vi "DownloadSettings.vi"() -> (1 "Yaxis":dbl[](array[numeric]), 2 "Xaxis":dbl[](array[numeric]), 3 "name":string)   [LabVIEW 2020]
panel:
  in  "Path":path
  in  "Multiplty (Iteration time)":dbl
  in  "OK":bool
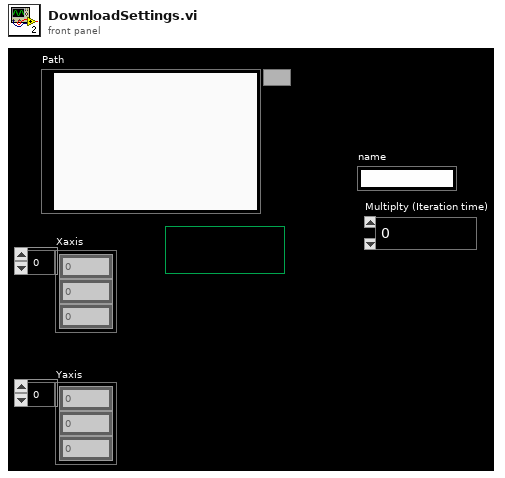
[diagram p1: front panel]
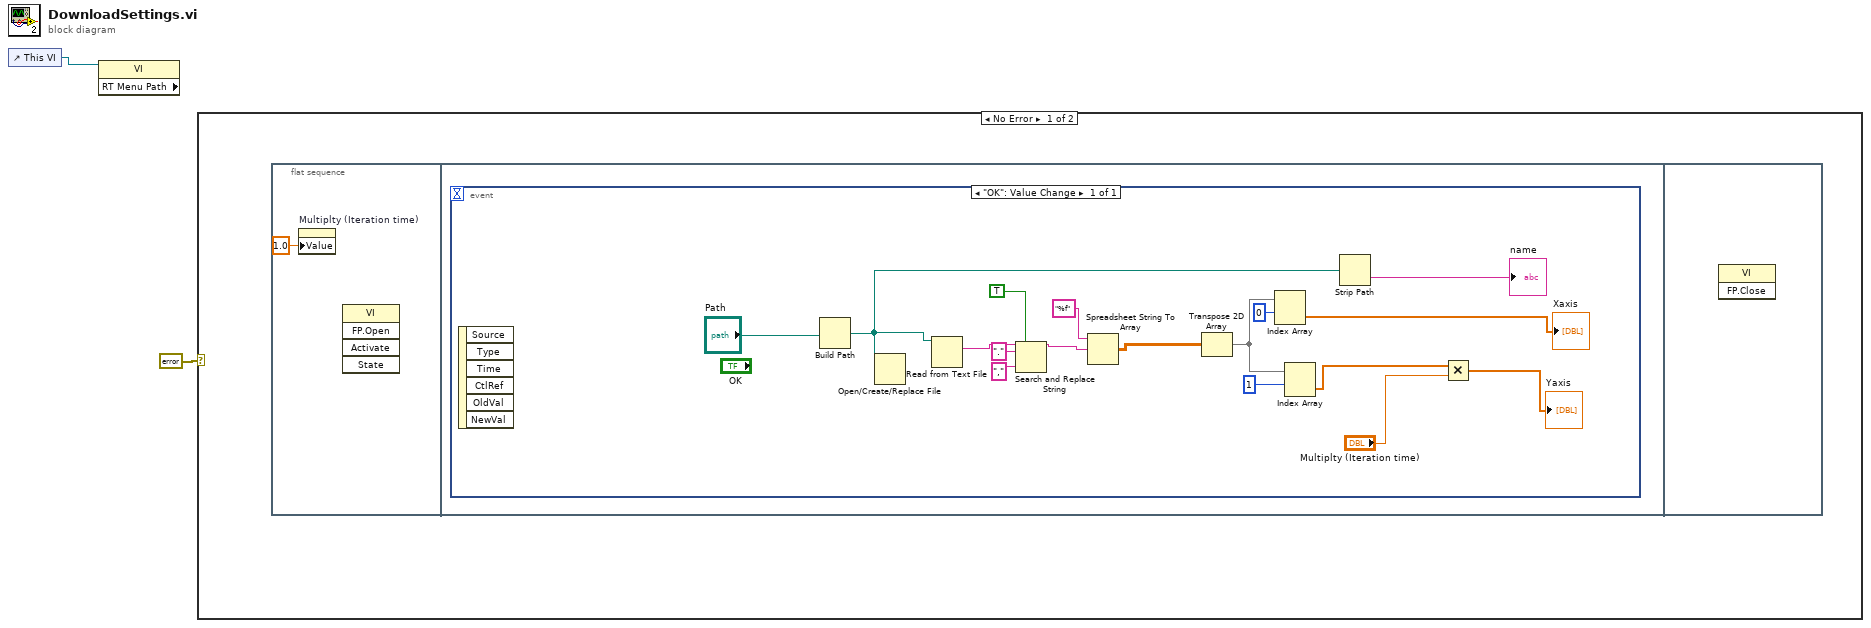
[diagram p0: block diagram]
diagram:
  n1 = control-ref of="This VI"() -> (w1:refnum<vi>)
  n2 = property class="VI" props=["RT Menu Path"](reference=w1) -> ()  [unwired: 1 in, 3 out]
  n3 = case shown="No Error" errorcluster {"status"=FALSE, "code"=0, "source"=""} ("error constant") {
    frame No Error {
      n4 = flat-sequence {
        frame #0 {
          n5 = property on="Multiplty (Iteration time)" class="DigNum (strict)"("Value"=1.0 ("Multiplty (Iteration time)")) -> ()  [unwired: 2 in, 2 out]
          n6 = invoke class="VI" method="FP.Open"() -> ()  [unwired: 5 in, 5 out]
        }
        frame #1 {
          n7 = event shown="[0] \"OK\": Value Change" {
            selector: _ -> [_]
            dyn-events: _ -> [_]
            timeout: _ -> [_]
            event "OK": Value Change {
              n8 = event-data() -> ()  [unwired: 1 in, 6 out]
              n9 = Build Path(name or relative path="Path") -> (appended path=w10:path)  [unwired: 1 in]
              n10 = Open/Create/Replace File(file path (use dialog)=w10) -> ()  [unwired: 5 in, 3 out]
              n11 = Read from Text File(file (use dialog)=w10) -> (text=w16:string)  [unwired: 3 in, 3 out]
              n12 = Search and Replace String(replace all?=TRUE ("replace all? (F)"), input string=w16, search string=".", replace string="," ("replace string (\"\")")) -> (result string=w12:string)  [unwired: 4 in, 3 out]
              n13 = Spreadsheet String To Array(format string="%f", spreadsheet string=w12) -> (array=w11:dbl[][])  [unwired: 2 in]
              n14 = Transpose 2D Array(2D array=w11) -> (transposed array=w18:dbl[][])
              n15 = Index Array(array=w18, index (row)=0) -> (element=→"Xaxis":dbl[])  [unwired: 1 in]
              n16 = Index Array(array=w18, index (row)=1) -> (element=w9:dbl[])  [unwired: 1 in]
              n17 = Strip Path(path=w10) -> (name=→"name":string)  [unwired: 1 out]
              n18 = Multiply(x=w9, y="Multiplty (Iteration time)") -> (x*y=→"Yaxis":dbl[])
            }
          }
        }
        frame #2 {
          n19 = invoke class="VI" method="FP.Close"() -> ()  [unwired: 3 in, 3 out]
        }
      }
    }
    frame Error {
    }
  }
